vi "Read Variant (sta prop).vi"(8 "error in (no error)":errorcluster, 11 "Test Object in":refnum<class "Test Object.lvclass">) -> (0 "error out":errorcluster, 2 "Variant":variant, 3 "Test Object out":refnum<class "Test Object.lvclass">)   [LabVIEW 2015, in "Test Object.lvclass"]
uses:
  Test Object.lvclass
  Test Object.lvclass/Test Object.ctl
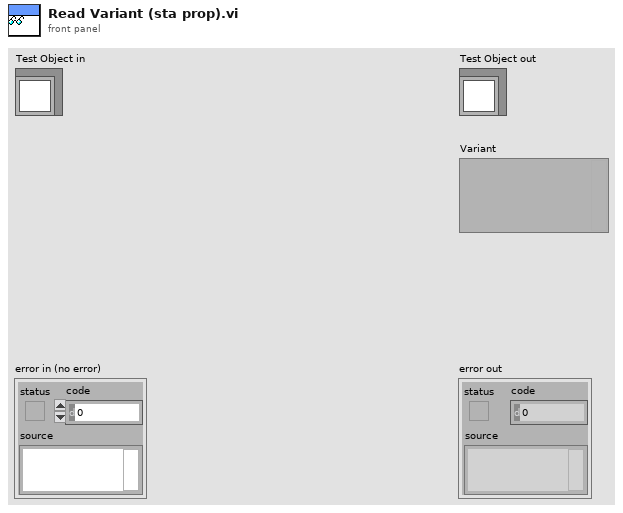
[diagram p1: front panel]
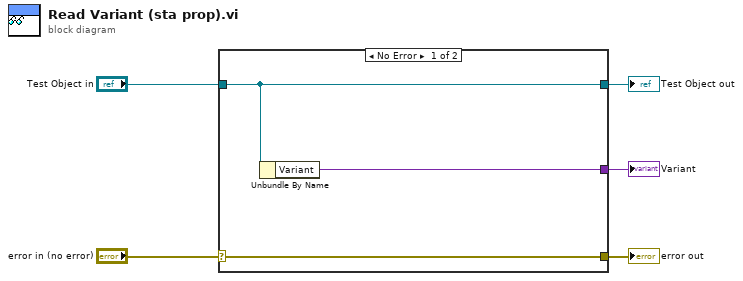
[diagram p0: block diagram]
diagram:
  n1 = case shown="No Error" "error in (no error)" {
    selector: "error in (no error)" -> [w8 w9]
    tunnel: [w8 w9] -> w4
    tunnel: [w7 w10] -> w2
    tunnel: "Test Object in" -> [w7 w10]
    tunnel: [w6 _] -> w1
    frame No Error {
      n2 = Unbundle By Name(w7) -> ("Variant"=w6:variant)
    }
    frame Error {
    }
  }
  "error out" <- w4
  "Test Object out" <- w2
  "Variant" <- w1
